vi "Write Grow Info.vi"(5 "Grow Info":T1, 9 "Control in":refnum<class "Control.lvclass">) -> (3 "Control out":refnum<class "Control.lvclass">)   [LabVIEW 2014, in "Raspberry Pi Compatible Compiler for LabVIEW.lvlib" / "Control.lvclass"]
uses:
  Control.lvclass
  Control.lvclass/Control.ctl
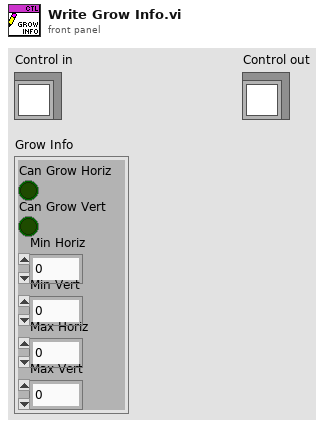
[diagram p1: front panel]
types:
  T1 = cluster{"Can Grow Horiz":bool, "Can Grow Vert":bool, "Min Horiz":i16, "Min Vert":i16, "Max Horiz":i16, "Max Vert":i16}
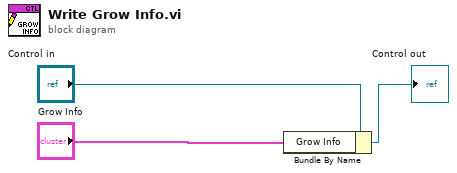
[diagram p0: block diagram]
diagram:
  n1 = Bundle By Name(cluster="Control in", "Grow Info"="Grow Info") -> (→"Control out":refnum<class "Control.lvclass">)
